vi "read_bytes.vi"(7 "read mode":T1(ring), 8 "error in (no error)":errorcluster, 9 "timeout (ms)":i32=-1, 10 "bytes to read":i32, 11 "Connection in":refnum<class "Connection.lvclass">) -> (0 "error out":errorcluster, 1 "data out":string, 2 "timeout?":bool, 3 "Connection out":refnum<class "Connection.lvclass">)   [LabVIEW 2019, in "Socket API.lvlib" / "Connection.lvclass"]
uses:
  Connection.lvclass
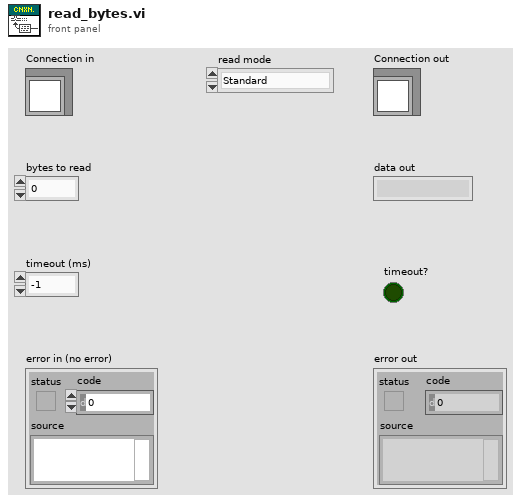
[diagram p1: front panel]
types:
  T1 = enum16{"Standard", "Buffered", "CRLF", "Immediate"}
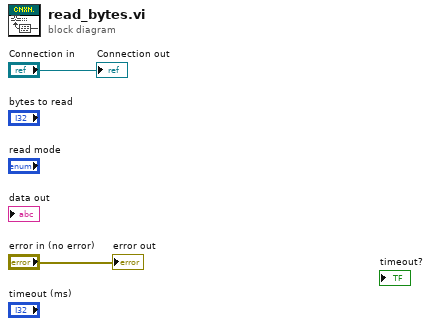
[diagram p0: block diagram]
diagram:
  "error out" <- "error in (no error)"
  "Connection out" <- "Connection in"
